vi "DELETEConvert Time Datatype string to enum.vi"(11 "Datatype":string) -> (3 "Time Datatype":T1)   [LabVIEW 2019]
uses:
  Typedefs/Time.Datatype--enum.ctl
  LV-Data.PGSQL.lvclass
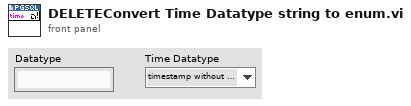
[diagram p1: front panel]
types:
  T1 = typedef "LV-Data.PGSQL.lvclass/Time.Datatype--enum.ctl" = enum16{"timestamp without time zone", "timestamp with time zone"}
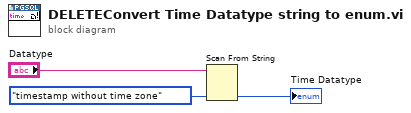
[diagram p0: block diagram]
diagram:
  n1 = Scan From String(input string="Datatype", default 1=Time.Datatype--enum."timestamp without time zone" ("Time Datatype")) -> (output 1=→"Time Datatype":T1)  [unwired: 3 in, 3 out]
